vi "Tree.vi"   [LabVIEW 2019, in "Control Experiment.lvclass"]
uses:
  Control Experiment.lvclass
  <userlib>/LevyLab/Krohn Hite 7008/Instrument.KH7008.lvclass
  <userlib>/LevyLab/Lockin-Multichannel/Instrument.Lockin/Instrument.Lockin.lvclass
  Typedefs/Instrument--enum.ctl
  SweepControl/SweepControl.lvclass
  Transport/Transport.lvclass
types:
  T1 = typedef "Control Experiment.lvclass/Instrument--enum.ctl" = enum16{"----- AFM/EBL -----", "AGILENT", "CYPHER", "Gemini2", "JEOL", "MFP3D", "----- Cryostat -----", "CF900", "DR200", "MNK", "PPMS (simulated)", "PPMS 1", "PPMS 2", "PPMS 3", "----- Optics -----", "THz 1 (Element 2/Montana)", "THz 2 (Tsunami/Janis)"}
  T2 = typedef "Control Experiment.lvclass/Instruments--cluster.ctl" = cluster{"KH7008":refnum<class "Instrument.KH7008.lvclass">[], "Lockin":refnum<class "Instrument.Lockin.lvclass">, "Temperature":refnum<class "Instrument.Cryostat.lvclass">, "Magnet":refnum<class "Instrument.Cryostat.lvclass">, "Rotator":refnum<class "Instrument.Cryostat.lvclass">, "Level":refnum<class "Instrument.Cryostat.lvclass">, "Capacitance Bridge":refnum<class "Instrument.CBridge.lvclass">, "Delay Line":refnum<class "Instrument.DelayLine.lvclass">, "Strain Cell":refnum<class "Instrument.Strain.lvclass">, "VNA":refnum<class "Instrument.VNA.lvclass">, "Voltage Source":refnum<class "Instrument.VSource.lvclass">}
  T3 = cluster{"key-value":cluster{"key":string, "value":dbl}}[]
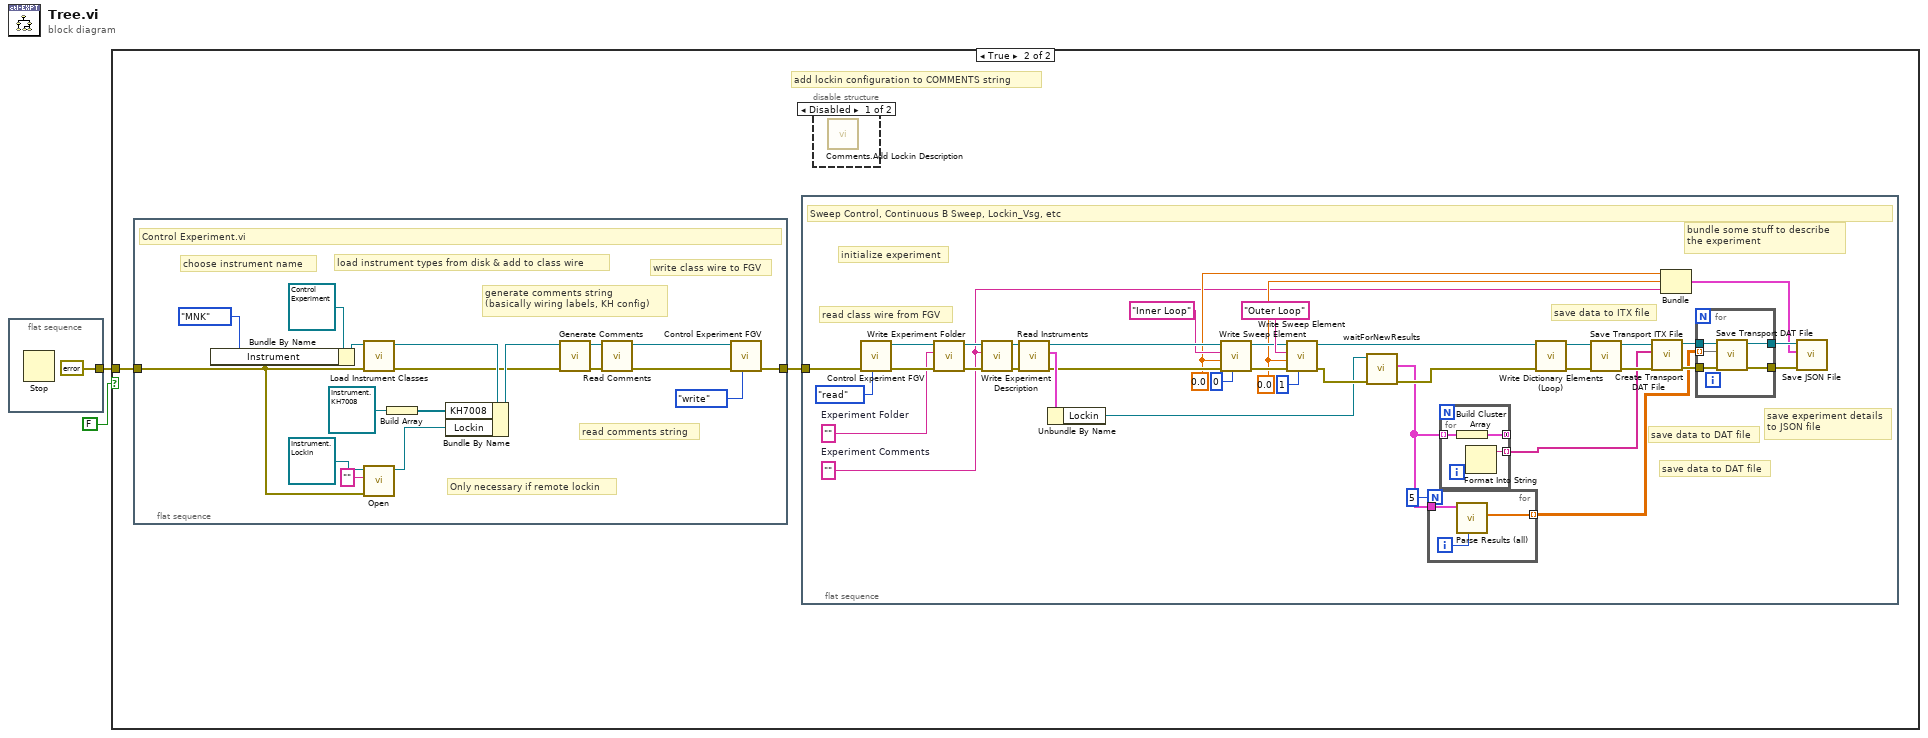
[diagram p0: block diagram]
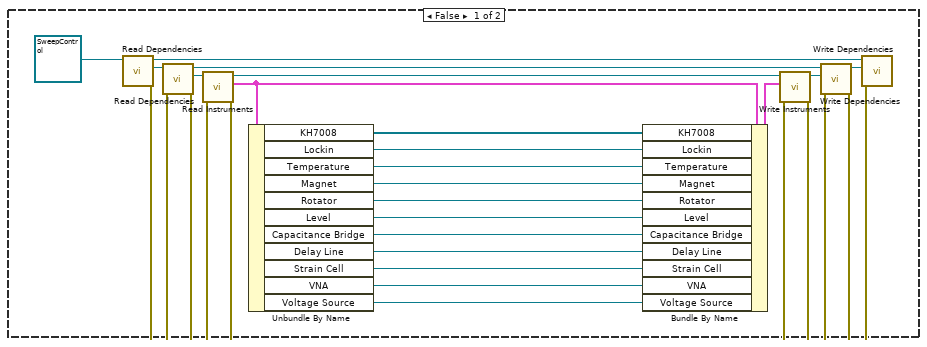
[diagram p2: hidden frame]
diagram:
  n1 = flat-sequence {
    tunnel: [errorcluster {"status"=FALSE, "code"=0, "source"=""} ("error in (no error)")] -> w2
    frame #0 {
      n2 = Stop() -> ()  [unwired: 1 in]
    }
  }
  n3 = case shown="True" FALSE {
    tunnel: w2 -> [_ w31]
    frame False {
      n4 = call "Read Dependencies.vi"("SweepControl in"=refnum<class "SweepControl.lvclass"> refnum ("SweepControl.lvclass")) -> ("error out"=w9:errorcluster, "Transport"=w28:refnum<class "Transport.lvclass">, "SweepControl out"=w26:refnum<class "SweepControl.lvclass">)  [unwired: 8 in]
      n5 = call "Read Dependencies.vi"("error in (no error)"=w9, "Transport"=w28) -> ("error out"=w8:errorcluster, "C.E."=w25:refnum<class "Control Experiment.lvclass">, "Transport"=w24:refnum<class "Transport.lvclass">)  [unwired: 7 in]
      n6 = call "Read Instruments.vi"("error in (no error)"=w8, "Control Experiment in"=w25) -> ("error out"=w4:errorcluster, "Instruments"=w22:T2, "Control Experiment out"=w5:refnum<class "Control Experiment.lvclass">)  [unwired: 7 in]
      n7 = Unbundle By Name(w22) -> ("KH7008"=w20:refnum<class "Instrument.KH7008.lvclass">[], "Lockin"=w19:refnum<class "Instrument.Lockin.lvclass">, "Temperature"=w18:refnum<class "Instrument.Cryostat.lvclass">, "Magnet"=w17:refnum<class "Instrument.Cryostat.lvclass">, "Rotator"=w16:refnum<class "Instrument.Cryostat.lvclass">, "Level"=w15:refnum<class "Instrument.Cryostat.lvclass">, "Capacitance Bridge"=w14:refnum<class "Instrument.CBridge.lvclass">, "Delay Line"=w13:refnum<class "Instrument.DelayLine.lvclass">, "Strain Cell"=w12:refnum<class "Instrument.Strain.lvclass">, "VNA"=w11:refnum<class "Instrument.VNA.lvclass">, "Voltage Source"=w10:refnum<class "Instrument.VSource.lvclass">)
      n8 = Bundle By Name(cluster=w22, "KH7008"=w20, "Lockin"=w19, "Temperature"=w18, "Magnet"=w17, "Rotator"=w16, "Level"=w15, "Capacitance Bridge"=w14, "Delay Line"=w13, "Strain Cell"=w12, "VNA"=w11, "Voltage Source"=w10) -> (w21:T2)
      n9 = call "Write Instruments.vi"("error in (no error)"=w4, "Instruments"=w21, "Control Experiment in"=w5) -> ("error out"=w7:errorcluster, "Control Experiment out"=w23:refnum<class "Control Experiment.lvclass">)  [unwired: 7 in]
      n10 = call "Write Dependencies.vi"("error in (no error)"=w7, "Control Experiment"=w23, "Transport in"=w24) -> ("error out"=w6:errorcluster, "Transport out"=w29:refnum<class "Transport.lvclass">)  [unwired: 7 in]
      n11 = call "Write Dependencies.vi"("error in (no error)"=w6, "Transport"=w29, "SweepControl in"=w26) -> ()  [unwired: 7 in, 2 out]
    }
    frame True {
      # "add lockin configuration to COMMENTS string"
      n12 = flat-sequence {
        tunnel: w31 -> [w88]
        tunnel: [w87] -> w30
        frame #0 {
          # "choose instrument name"
          # "Only necessary if remote lockin"
          # "write class wire to FGV"
          # "read comments string"
          # "generate comments string\n(basically wiring labels, KH config)"
          # "load instrument types from disk & add to class wire"
          # "Control Experiment.vi"
          n13 = Bundle By Name(cluster=refnum<class "Control Experiment.lvclass"> refnum ("Control Experiment.lvclass"), "Instrument"=Instrument--enum."MNK" ("Experiment.Instrument")) -> (w84:refnum<class "Control Experiment.lvclass">)
          n14 = call "Load Instrument Classes.vi"("error in (no error)"=w88, "Control Experiment.lvclass"=w84) -> ("error out"=w92:errorcluster, "Control Experiment out"=w94:refnum<class "Control Experiment.lvclass">)  [unwired: 8 in]
          n15 = call-dynamic "Open.vi"("error in (no error)"=w88, "address"="" ("Address"), "Instrument.Lockin in"=refnum<class "Instrument.Lockin.lvclass"> refnum ("Instruments.Lockin")) -> ("Instrument.Lockin out"=w96:refnum<class "Instrument.Lockin.lvclass">)  [unwired: 7 in, 1 out]
          n16 = Build Array(refnum<class "Instrument.KH7008.lvclass"> refnum ("Instruments.KH7008")) -> (w82:refnum<class "Instrument.KH7008.lvclass">[])
          n17 = Bundle By Name(cluster=w94, "KH7008"=w82, "Lockin"=w96) -> (w93:refnum<class "Control Experiment.lvclass">)
          n18 = call "Generate Comments.vi"("error in (no error)"=w92, "Control Experiment"=w93) -> ("error out"=w99:errorcluster, "Control Experiment out"=w98:refnum<class "Control Experiment.lvclass">)  [unwired: 6 in, 1 out]
          n19 = call "Read Comments.vi"("error in (no error)"=w99, "Control Experiment in"=w98) -> ("error out"=w91:errorcluster, "Control Experiment out"=w90:refnum<class "Control Experiment.lvclass">)  [unwired: 7 in, 1 out]
          n20 = call "Control Experiment FGV.vi"("Function"=enum16{"read", "write"}."write", "error in (no error)"=w91, "Control Experiment.lvclass"=w90) -> ("error out"=w87:errorcluster)  [unwired: 7 in, 1 out]
        }
      }
      n21 = flat-sequence {
        tunnel: w30 -> [w69]
        frame #0 {
          w42 = ""  # Experiment Comments
          w41 = ""  # Experiment Folder
          w43 = 0.0
          w44 = 0.0
          # "initialize experiment"
          # "save experiment details\nto JSON file"
          # "save data to DAT file"
          # "save data to DAT file"
          # "save data to ITX file"
          # "bundle some stuff to describe\nthe experiment"
          # "read class wire from FGV"
          # "Sweep Control, Continuous B Sweep, Lockin_Vsg, etc"
          n22 = call "Control Experiment FGV.vi"("Function"=enum16{"read", "write"}."read", "error in (no error)"=w69) -> ("error out"=w65:errorcluster, "Control Experiment.lvclass out"=w64:refnum<class "Control Experiment.lvclass">)  [unwired: 8 in]
          n23 = call "Write Experiment Folder.vi"("error in (no error)"=w65, "Experiment Folder"=w41, "Control Experiment in"=w64) -> ("error out"=w66:errorcluster, "Control Experiment out"=w67:refnum<class "Control Experiment.lvclass">)  [unwired: 7 in]
          n24 = call "Write Experiment Description.vi"("error in (no error)"=w66, "Experiment Description"=w42, "Control Experiment in"=w67) -> ("error out"=w63:errorcluster, "Control Experiment out"=w62:refnum<class "Control Experiment.lvclass">)  [unwired: 7 in]
          n25 = call "Read Instruments.vi"("error in (no error)"=w63, "Control Experiment in"=w62) -> ("error out"=w60:errorcluster, "Instruments"=w61:T2, "Control Experiment out"=w59:refnum<class "Control Experiment.lvclass">)  [unwired: 7 in]
          n26 = Unbundle By Name(w61) -> ("Lockin"=w40:refnum<class "Instrument.Lockin.lvclass">)
          n27 = call "Write Sweep Element.vi"("loop index"=0, "error in (no error)"=w60, "value"=w44, "key"="Inner Loop", "Control Experiment in"=w59) -> ("error out"=w53:errorcluster, "Control Experiment out"=w54:refnum<class "Control Experiment.lvclass">)  [unwired: 5 in]
          n28 = call "Write Sweep Element.vi"("loop index"=1, "error in (no error)"=w53, "value"=w43, "key"="Outer Loop", "Control Experiment in"=w54) -> ("error out"=w52:errorcluster, "Control Experiment out"=w39:refnum<class "Control Experiment.lvclass">)  [unwired: 5 in]
          n29 = call <userlib>:"waitForNewResults.vi"("error in (no error)"=w52, "Instrument.Lockin in"=w40) -> ("error out"=w37:errorcluster, "Results (Dictionary)"=w34:cluster{"key":string, "value":dbl}[])  [unwired: 7 in, 1 out]
          n30 = for {
            N: 5 -> [_]
            tunnel: w34 -> [w72]
            tunnel: [w71] -> w33 mode=indexing
            i -> [w70]
            n31 = call <userlib>:"Parse Results (all).vi"("Type"=w70, "Results (Dictionary)"=w72) -> ("Data"=w71:dbl[])  [unwired: 6 in, 3 out]
          }
          n32 = for {
            tunnel: w34 -> [w81] mode=indexing
            tunnel: [w80] -> _ mode=concatenating
            tunnel: [w78] -> w35 mode=indexing
            i -> [w79]
            n33 = Build Cluster Array(w81) -> (w80:T3)
            n34 = Format Into String(w79) -> (resulting string=w78:string)  [unwired: 3 in, 1 out]
          }
          n35 = call "Write Dictionary Elements (Loop).vi"("error in (no error)"=w37, "Control Experiment in"=w39) -> ("error out"=w36:errorcluster, "Control Experiment out"=w38:refnum<class "Control Experiment.lvclass">)  [unwired: 8 in]
          n36 = call "Save Transport ITX File.vi"("error in (no error)"=w36, "Control Experiment in"=w38) -> ("error out"=w50:errorcluster, "Control Experiment out"=w51:refnum<class "Control Experiment.lvclass">)  [unwired: 8 in]
          n37 = call "Create Transport DAT File.vi"("error in (no error)"=w50, "Wavenames"=w35, "Control Experiment in"=w51) -> ("error out"=w48:errorcluster, "Control Experiment out"=w49:refnum<class "Control Experiment.lvclass">)  [unwired: 7 in]
          n38 = Bundle(w44, w43, "Experiment Comments"=w42) -> (w45:cluster{dbl, dbl, "Experiment Comments":string})  [unwired: 1 in]
          n39 = for {
            tunnel: w33 -> [w73] mode=indexing
            tunnel: w49 -> [w77]
            tunnel: [w75] -> w47
            tunnel: w48 -> [w76]
            tunnel: [w74] -> w46
            n40 = call "Save Transport DAT File.vi"("error in (no error)"=w76, "Data (Row)"=w73, "Control Experiment in"=w77) -> ("error out"=w74:errorcluster, "Control Experiment out"=w75:refnum<class "Control Experiment.lvclass">)  [unwired: 7 in]
          }
          n41 = call "Save JSON File.vi"("error in (no error)"=w46, "Data"=w45, "Control Experiment in"=w47) -> ()  [unwired: 8 in, 1 out]
        }
      }
      n42 = disable-structure shown="Disabled" {
        frame Disabled {
          n43 = call "Comments.Add Lockin Description.vi"() -> ()  [unwired: 9 in, 2 out]
        }
        frame Enabled {
        }
      }
    }
  }
